vi "DisplayDataOfNoDuplicationTo2DListCtrl.vi"(8 "display string":string="DMM", 9 "check name":string="DMM", 10 "check column index":u32, 11 "ArrayRef in":refnum<vi>) -> (3 "ArrayRef out":refnum<vi>)   [LabVIEW 2018, in "Library-Ctrl.lvlib"]
uses:
  Library-Ctrl.lvlib
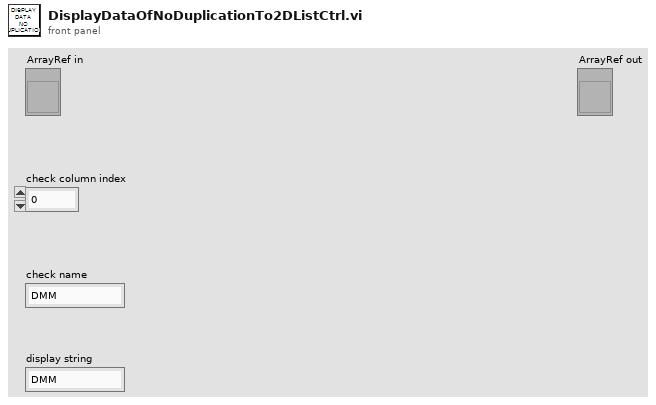
[diagram p1: front panel]
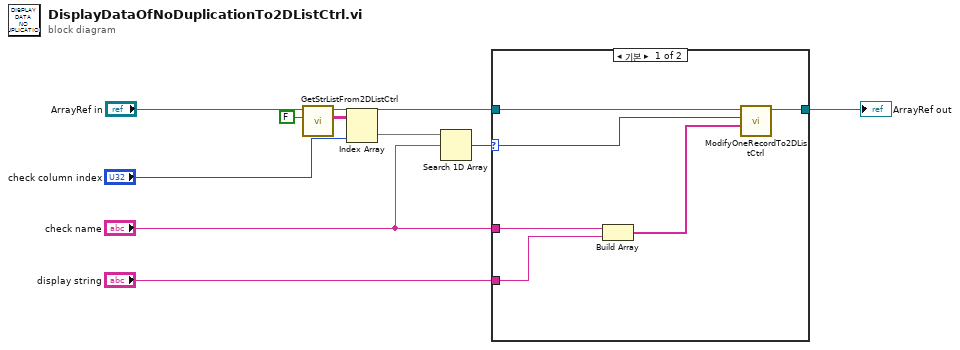
[diagram p0: block diagram]
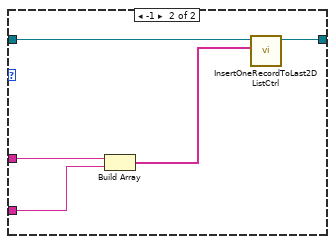
[diagram p2: hidden frame]
diagram:
  n1 = call "GetStrListFrom2DListCtrl.vi"("include index?"=FALSE, "ref 2D list in"="ArrayRef in") -> ("result"=w9:string[][], "ref 2D list out"=w5:refnum<vi>)  [unwired: 8 in]
  n2 = Index Array(array=w9, index (col)="check column index") -> (element=w7:string[])  [unwired: 1 in]
  n3 = Search 1D Array(1D array=w7, element="check name") -> (index of element=w6:i32)  [unwired: 1 in]
  n4 = case shown="기본" w6 {
    selector: w6 -> [w15 _]
    tunnel: w5 -> [w16 w21]
    tunnel: "display string" -> [w13 w19]
    tunnel: "check name" -> [w14 w20]
    tunnel: [w11 w17] -> w2
    frame Default {
      n5 = Build Array(w14, w13) -> (w12:string[])
      n6 = call "ModifyOneRecordTo2DListCtrl.vi"(9:w12, "arr data"=w15, "multiple list in"=w16) -> ("multiple list out"=w11:refnum<vi>)  [unwired: 8 in]
    }
    frame -1 {
      n7 = Build Array(w20, w19) -> (w18:string[])
      n8 = call "InsertOneRecordToLast2DListCtrl.vi"("arr data"=w18, "testcaselist in"=w21) -> ("testcaselist out"=w17:refnum<vi>)  [unwired: 9 in]
    }
  }
  "ArrayRef out" <- w2
